vi "Bearing Given Two points.vi"(10 "End Point":T1 {"Latitude" format="%#_10g"; "Longitude" format="%#_10g"}, 11 "Origin Point":T1 {"Latitude" format="%#_10g"; "Longitude" format="%#_10g"}) -> (2 "True Angle":dbl, 3 "Bearing (True North)":dbl)   [LabVIEW 2014]
uses:
  Controls/PointLatLon.ctl
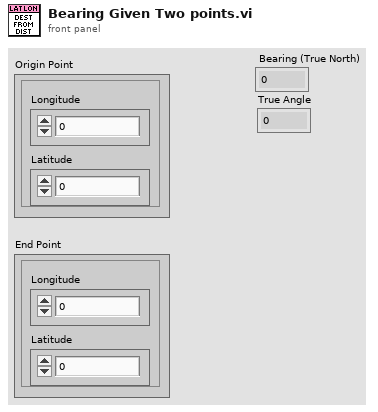
[diagram p1: front panel]
types:
  T1 = typedef "PointLatLon.ctl" = cluster{"Longitude":dbl, "Latitude":dbl}
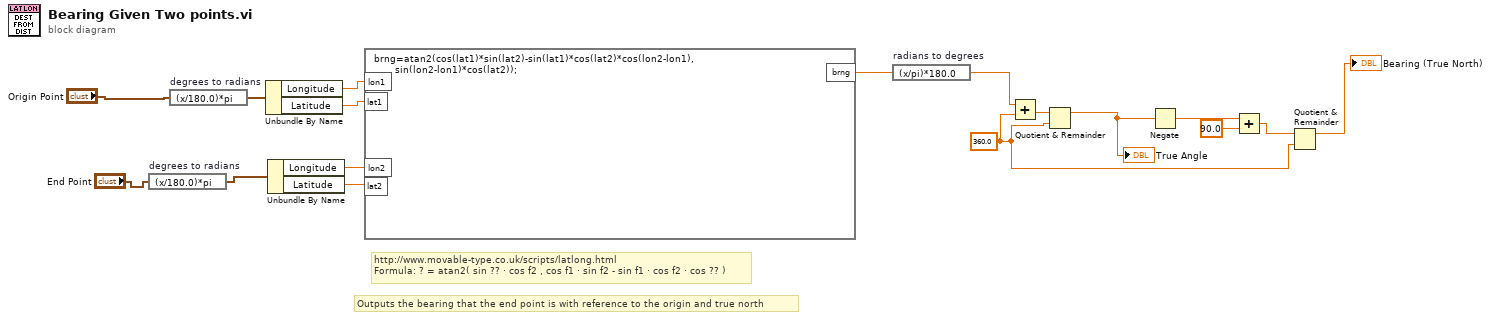
[diagram p0: block diagram]
diagram:
  w2 = 360.0 ("y")
  # "Outputs the bearing that the end point is with reference to the origin and true north"
  # "http://www.movable-type.co.uk/scripts/latlong.html\nFormula:\t? = atan2( sin ?? · cos f2 , cos f1 · sin f2 - sin f1 · cos f2 · cos ?? )"
  n1 = expression code="(x/180.0)*pi" "degrees to radians"("End Point") -> (w14:T1)
  n2 = expression code="(x/180.0)*pi" "degrees to radians"("Origin Point") -> (w17:T1)
  n3 = Unbundle By Name(w17) -> ("Longitude"=w15:dbl, "Latitude"=w16:dbl)
  n4 = Unbundle By Name(w14) -> ("Longitude"=w13:dbl, "Latitude"=w12:dbl)
  n5 = formula code="brng=atan2(cos(lat1)*sin(lat2)-sin(lat1)*cos(lat2)*cos(lon2-lon1), \n       sin(lon2-lon1)*cos(lat2));"("lon1"=w15, "lat1"=w16, "lon2"=w13, "lat2"=w12) -> ("brng"=w11:dbl)
  n6 = expression code="(x/pi)*180.0" "radians to degrees"(w11) -> (w10:dbl)
  n7 = Add(x=w10, y=w2) -> (x+y=w9:dbl)
  n8 = Quotient & Remainder(x=w9, y=w2) -> (x-y*floor(x/y)=w6:dbl)  [unwired: 1 out]
  "True Angle" <- w6
  n9 = Negate(x=w6) -> (-x=w5:dbl)
  n10 = Add(x=w5, y=90.0) -> (x+y=w3:dbl)
  n11 = Quotient & Remainder(x=w3, y=w2) -> (x-y*floor(x/y)=→"Bearing (True North)":dbl)  [unwired: 1 out]
